vi "ProcessButtonPressed.vi"(6 "Queue in":refnum<queue>, 7 "On Delay Time\nSeconds":dbl, 8 "Time":dbl=-1.0, 9 "ButtonNumber":i32, 10 "ElapsedTime":dbl, 11 "RawButtonInput":bool) -> ()   [LabVIEW 2025]
uses:
  ButtonInfoTypeDef.ctl
  <vilib>/Rock Robotics/WPI/ThirdParty/JAS_Junk/TrajLib/Timer_New.vi
  <vilib>/Utility/semaphor.llb/Obtain Semaphore Reference.vi
  <vilib>/Rock Robotics/WPI/ThirdParty/JAS_Junk/TrajLib/Timer_Reset.vi
  <vilib>/Rock Robotics/WPI/ThirdParty/JAS_Junk/TrajLib/Timer_Start.vi
  <vilib>/Rock Robotics/WPI/ThirdParty/JAS_Junk/TrajLib/Timer_Stop.vi
  <vilib>/Rock Robotics/WPI/ThirdParty/JAS_Junk/TrajLib/Timer_HasPeriodPassedOnce.vi
  <vilib>/Rock Robotics/WPI/ThirdParty/JAS_Junk/TrajLib/Trajectory_Library.lvlib
  Robot Global Data.vi
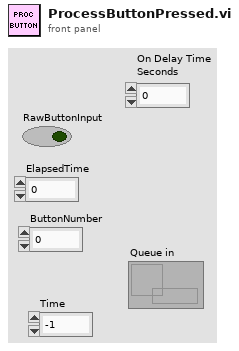
[diagram p1: front panel]
types:
  T1 = typedef "ButtonInfoTypeDef.ctl" = cluster{"ElapsedTime":dbl, "ButtonNumber":i32}
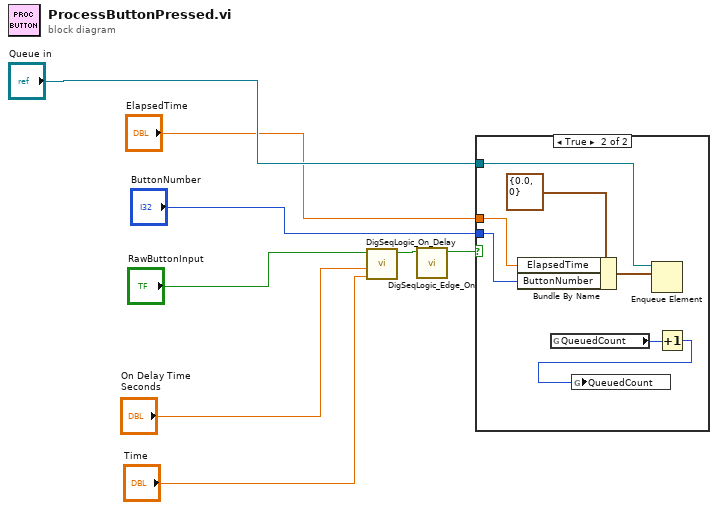
[diagram p0: block diagram]
diagram:
  n1 = call <vilib>:"DigSeqLogic_On_Delay.vi"("Time"="Time", "Delay"="On Delay Time\nSeconds", "Input"="RawButtonInput") -> ("Output"=w4:bool)  [unwired: 7 in, 1 out]
  n2 = call <vilib>:"DigSeqLogic_Edge_On.vi"("Input"=w4) -> ("On Edge"=w5:bool)  [unwired: 10 in]
  n3 = case shown="True" w5 {
    tunnel: "ElapsedTime" -> [_ w14]
    tunnel: "ButtonNumber" -> [_ w13]
    tunnel: "Queue in" -> [_ w12]
    frame False {
    }
    frame True {
      n4 = Bundle By Name(cluster=T1 {"ElapsedTime"=0.0, "ButtonNumber"=0} ("ButtonPressedInfo"), "ElapsedTime"=w14, "ButtonNumber"=w13) -> (w11:T1)
      n5 = global read "Robot Global Data.vi" "QueuedCount"() -> (w10:i32)
      n6 = Enqueue Element(queue=w12, element=w11) -> ()  [unwired: 2 in, 3 out]
      n7 = Increment(x=w10) -> (x+1=w9:i32)
      n8 = global write "Robot Global Data.vi" "QueuedCount"(w9) -> ()
    }
  }
